vi "BCU参数读取-Auto.vi"(8 "CAN端口":u16(ring), 9 "设备索引号":u16(ring), 10 "CAN卡类型":u32(ring)=21, 11 "Myindex":dbl=1.0) -> (3 "成功":bool)   [LabVIEW 2013] (continued)
                          n1972 = global write "EV05全局变量1.vi" "流控帧 2"(FALSE ("流控帧 2")) -> ()
                          n1973 = global write "EV05全局变量1.vi" "输出数组"(i32[] []) -> ()
                          n1974 = local write "控制1"(FALSE ("控制1")) -> ()
                          n1975 = local write "消除"(FALSE ("消除")) -> ()
                        }
                      }
                    }
                    frame True {
                      # "写参数判定"
                      n1976 = And(x="控制1", y=w3317) -> (x .and. y?=w3314:bool)
                      n1977 = case shown="真" w3314 {
                        tunnel: w3316 -> [_ w3324]
                        tunnel: w3315 -> [_ w3321]
                        frame False {
                        }
                        frame True {
                          n1978 = call <vilib>:"Unset Busy.vi"() -> ()  [unwired: 2 in, 10 out]
                          n1979 = case shown="\"主板\", 默认" w3321 {
                            tunnel: [w3325 w3326] -> w3323
                            frame "主板", Default {
                              n1980 = local read "主板选项"() -> (w3325:string)
                            }
                            frame "从板" {
                              n1981 = local read "从板选项"() -> (w3326:string)
                            }
                          }
                          n1982 = control-ref of="结果"() -> (w3322:refnum<vi>)
                          n1983 = call "输入数据判定.vi"("主从选择"=w3321, "主板选项"=w3323, "进度引用"=w3322, "错误代码"=w3324) -> ()  [unwired: 3 in, 5 out]
                          n1984 = global write "EV05全局变量1.vi" "流控帧 2"(FALSE ("流控帧 2")) -> ()
                          n1985 = local write "控制1"(FALSE ("控制1")) -> ()
                          n1986 = local write "消除"(FALSE ("消除")) -> ()
                        }
                      }
                      n1987 = global write "EV05全局变量1.vi" "输出数组"(i32[] []) -> ()
                    }
                  }
                }
                frame "版本读取" {
                  n1988 = local read "命令序号"() -> (w3327:u8)
                  n1989 = local read "从板板号"() -> (w3330:u8)
                  n1990 = local read "控制1"() -> (w3331:bool)
                  n1991 = call "多帧接收机制(EV05).vi"("can卡类型"=w3338, "设备索引号"=w3337, "CAN端口"=w3336, "VCI_Receive"=w3335, "命令"=w3334, "板号"=w3330, "命令序号"=w3327) -> ("错误信号"=w3328:bool, "输出数组"=w3339:u8[], "读错误代码"=w3329:u8[], "结束信号"=w3333:bool)  [unwired: 3 in, 6 out]
                  n1992 = And(x=w3331, y=w3333) -> (x .and. y?=w3332:bool)
                  n1993 = case shown="真" w3332 {
                    tunnel: w3339 -> [_ w3347]
                    tunnel: w3327 -> [_ w3346]
                    tunnel: w3334 -> [_ w3345]
                    tunnel: w3329 -> [_ w3341]
                    tunnel: w3328 -> [_ w3340]
                    frame False {
                    }
                    frame True {
                      n1994 = case shown="假" w3340 {
                        tunnel: w3347 -> [w3351 _]
                        tunnel: w3346 -> [w3350 _]
                        tunnel: w3345 -> [w3349 _]
                        tunnel: w3341 -> [w3348 w3575]
                        frame False {
                          n1995 = case shown="89" w3349 {
                            tunnel: w3350 -> [_ w3354]
                            tunnel: w3351 -> [_ w3353]
                            tunnel: w3348 -> [_ _]
                            frame 0, Default {
                            }
                            frame 137 {
                              n1996 = case shown="1" w3354 {
                                tunnel: w3353 -> [_ w3382 w3426 w3446 w3573]
                                frame 0, Default {
                                }
                                frame 1 {
                                w3364 = "." ("字符串")
                                n1997 = Array Subset(array=w3382, index=0 ("索引"), length=14 ("长度")) -> (w3395:u8[])
                                n1998 = Index Array(array=w3382, index=14 ("索引")) -> (element=w3385:u8)
                                n1999 = Index Array(array=w3382, index #1=15 ("索引"), index #2=16 ("索引")) -> (element #1=w3391:u8, element #2=w3392:u8)
                                n2000 = Index Array(array=w3382, index #1=17 ("索引"), index #2=18 ("索引")) -> (element #1=w3386:u8, element #2=w3387:u8)
                                n2001 = call "数组去零.vi"("输入"=w3395) -> ("输出"=w3370:dbl[])
                                n2002 = Join Numbers(hi=w3386, lo=w3387) -> ((hi.lo)=w3383:u16)
                                n2003 = Join Numbers(hi=w3391, lo=w3392) -> ((hi.lo)=w3384:u16)
                                n2004 = Number To Decimal String(number=w3385) -> (decimal integer string=w3377:string)  [unwired: 1 out]
                                n2005 = Byte Array To String(unsigned byte array=w3370) -> (string=w3369:string)
                                n2006 = Number To Decimal String(number=w3383) -> (decimal integer string=w3365:string)  [unwired: 1 out]
                                n2007 = Number To Decimal String(number=w3384) -> (decimal integer string=w3376:string)  [unwired: 1 out]
                                n2008 = Array Subset(array=w3382, index=21 ("索引"), length=7 ("长度")) -> (w3379:u8[])
                                n2009 = Concatenate Strings("V" ("字符串"), w3377, w3364, w3376, w3364, w3365) -> (w3374:string)
                                n2010 = call "数组去零.vi"("输入"=w3379) -> ("输出"=w3362:dbl[])
                                n2011 = Byte Array To String(unsigned byte array=w3362) -> (string=w3360:string)
                                n2012 = call <vilib>:"Space Constant.vi"() -> ("String"=w3361:string)
                                n2013 = Equal?(x=w3360, y=w3361) -> (x = y?=w3366:bool)
                                n2014 = Concatenate Strings("-" ("字符串"), w3360) -> (w3367:string)
                                n2015 = Select(t=w3361, s=w3366, f=w3367) -> (s? t:f=w3363:string)
                                n2016 = Concatenate Strings(w3369, "-" ("字符串"), w3374, w3363) -> (w3356:string)
                                n2017 = local read "项目软件版本"() -> (w3358:string[])
                                n2018 = local read "从板板号"() -> (w3355:u8)
                                n2019 = local write "项目软件版本号"(w3356) -> ()
                                n2020 = Replace Array Subset(array=w3358, new element=w3356, index=w3355) -> (w3357:string[])
                                n2021 = control-ref of="结果"() -> (w3373:refnum<vi>)
                                n2022 = local write "项目软件版本"(w3357) -> ()
                                n2023 = Build Array("项目软件版本     读取完成" ("读取结果")) -> (w3371:string[])
                                n2024 = call "表格编辑(版本读取).vi"("新元素/子数组"=w3371, "活动单元格:单元格背景色"=u32 6618880, "MCListbox引用句柄"=w3373) -> ()  [unwired: 9 out]
                                }
                                frame 2 {
                                w3409 = ""
                                w3406 = "." ("字符串")
                                n2025 = Array Subset(array=w3426, index=0 ("索引"), length=14 ("长度")) -> (w3414:u8[])
                                n2026 = Index Array(array=w3426, index=14 ("索引")) -> (element=w3429:u8)
                                n2027 = Index Array(array=w3426, index #1=15 ("索引"), index #2=16 ("索引")) -> (element #1=w3435:u8, element #2=w3436:u8)
                                n2028 = Index Array(array=w3426, index #1=17 ("索引"), index #2=18 ("索引")) -> (element #1=w3430:u8, element #2=w3431:u8)
                                n2029 = Join Numbers(hi=w3430, lo=w3431) -> ((hi.lo)=w3427:u16)
                                n2030 = Join Numbers(hi=w3435, lo=w3436) -> ((hi.lo)=w3428:u16)
                                n2031 = Number To Decimal String(number=w3427) -> (decimal integer string=w3407:string)  [unwired: 1 out]
                                n2032 = call "数组去零.vi"("输入"=w3414) -> ("输出"=w3413:dbl[])
                                n2033 = Number To Decimal String(number=w3429) -> (decimal integer string=w3421:string)  [unwired: 1 out]
                                n2034 = Number To Decimal String(number=w3428) -> (decimal integer string=w3420:string)  [unwired: 1 out]
                                n2035 = Array Subset(array=w3426, index=21 ("索引"), length=7 ("长度")) -> (w3423:u8[])
                                n2036 = Byte Array To String(unsigned byte array=w3413) -> (string=w3408:string)
                                n2037 = call "数组去零.vi"("输入"=w3423) -> ("输出"=w3405:dbl[])
                                n2038 = Concatenate Strings("V" ("字符串"), w3421, w3406, w3420, w3406, w3407) -> (w3418:string)
                                n2039 = Byte Array To String(unsigned byte array=w3405) -> (string=w3403:string)
                                n2040 = Equal?(x=w3409, y=w3403) -> (x = y?=w3410:bool)
                                n2041 = Concatenate Strings("-" ("字符串"), w3403) -> (w3411:string)
                                n2042 = Select(t=w3409, s=w3410, f=w3411) -> (s? t:f=w3404:string)
                                n2043 = Concatenate Strings(w3408, "-" ("字符串"), w3418, w3404) -> (w3399:string)
                                n2044 = local read "平台软件版本"() -> (w3401:string[])
                                n2045 = local read "从板板号"() -> (w3398:u8)
                                n2046 = local write "平台软件版本号"(w3399) -> ()
                                n2047 = Replace Array Subset(array=w3401, new element=w3399, index=w3398) -> (w3400:string[])
                                n2048 = control-ref of="结果"() -> (w3416:refnum<vi>)
                                n2049 = local write "平台软件版本"(w3400) -> ()
                                n2050 = Build Array("平台软件版本     读取完成" ("读取结果")) -> (w3415:string[])
                                n2051 = call "表格编辑(版本读取).vi"("新元素/子数组"=w3415, "活动单元格:单元格背景色"=u32 6618880, "MCListbox引用句柄"=w3416) -> ()  [unwired: 1 in, 8 out]
                                }
                                frame 3 {
                                n2052 = Index Array(array=w3446, index #1=0 ("索引"), index #2=1 ("索引")) -> (element #1=w3442:u8, element #2=w3443:u8)
                                n2053 = Join Numbers(hi=w3442, lo=w3443) -> ((hi.lo)=w3441:u16)
                                n2054 = case shown="99, 默认" w3441 {
                                tunnel: w3446 -> [w3449 _ w3483]
                                tunnel: w3441 -> [_ _ w3461]
                                frame 0 {
                                n2055 = Index Array(array=w3449, index #1=2 ("索引"), index #2=3 ("索引")) -> (element #1=w3453:u8, element #2=w3452:u8)
                                n2056 = Join Numbers(hi=w3453, lo=w3452) -> ((hi.lo)=w3448:u16)
                                n2057 = for {
                                N: w3448 -> [_]
                                tunnel: w3449 -> [w3458]
                                tunnel: [w3454] -> w3447 mode=indexing
                                i -> [w3457]
                                n2058 = Add(x=w3457, y=4) -> (x+y=w3455:i32)
                                n2059 = Index Array(array=w3458, index=w3455) -> (element=w3454:u8)
                                }
                                "MODEL号" <- w3447
                                }
                                frame 99, Default {
                                }
                                frame 1..40 {
                                w3466 = ""
                                w3487 = "." ("字符串")
                                n2060 = Array Subset(array=w3483, index=2 ("索引"), length=14 ("长度")) -> (w3472:u8[])
                                n2061 = Index Array(array=w3483, index=16 ("索引")) -> (element=w3495:u8)
                                n2062 = Index Array(array=w3483, index #1=17 ("索引"), index #2=18 ("索引")) -> (element #1=w3501:u8, element #2=w3502:u8)
                                n2063 = Index Array(array=w3483, index #1=19 ("索引"), index #2=20 ("索引")) -> (element #1=w3496:u8, element #2=w3497:u8)
                                n2064 = Join Numbers(hi=w3496, lo=w3497) -> ((hi.lo)=w3493:u16)
                                n2065 = Join Numbers(hi=w3501, lo=w3502) -> ((hi.lo)=w3494:u16)
                                n2066 = Number To Decimal String(number=w3461) -> (decimal integer string=w3481:string)  [unwired: 1 out]
                                n2067 = Number To Decimal String(number=w3495) -> (decimal integer string=w3489:string)  [unwired: 1 out]
                                n2068 = call "数组去零.vi"("输入"=w3472) -> ("输出"=w3471:dbl[])
                                n2069 = Number To Decimal String(number=w3494) -> (decimal integer string=w3488:string)  [unwired: 1 out]
                                n2070 = Number To Decimal String(number=w3493) -> (decimal integer string=w3486:string)  [unwired: 1 out]
                                n2071 = Byte Array To String(unsigned byte array=w3471) -> (string=w3473:string)
                                n2072 = Concatenate Strings("第" ("读取结果"), w3481, "模块" ("字符串"), "     读取完成" ("读取结果")) -> (w3474:string)
                                n2073 = Concatenate Strings("V" ("字符串"), w3489, w3487, w3488, w3487, w3486) -> (w3484:string)
                                n2074 = control-ref of="结果"() -> (w3477:refnum<vi>)
                                n2075 = Array Subset(array=w3483, index=23 ("索引"), length=7 ("长度")) -> (w3470:u8[])
                                n2076 = call "数组去零.vi"("输入"=w3470) -> ("输出"=w3465:dbl[])
                                n2077 = Byte Array To String(unsigned byte array=w3465) -> (string=w3462:string)
                                n2078 = Build Array(w3474) -> (w3476:string[])
                                n2079 = control-ref of="模块软件版本 2"() -> (w3478:refnum<vi>)
                                n2080 = local read "模块软件版本"() -> (w3479:T1)
                                n2081 = Equal?(x=w3466, y=w3462) -> (x = y?=w3467:bool)
                                n2082 = call "表格编辑(版本读取).vi"("新元素/子数组"=w3476, "活动单元格:单元格背景色"=u32 6618880, "MCListbox引用句柄"=w3477) -> ()  [unwired: 1 in, 8 out]
                                n2083 = Concatenate Strings("-" ("字符串"), w3462) -> (w3468:string)
                                n2084 = Select(t=w3466, s=w3467, f=w3468) -> (s? t:f=w3464:string)
                                n2085 = Concatenate Strings(w3473, "-" ("字符串"), w3484, w3464) -> (w3463:string)
                                n2086 = case shown="30" w3461 {
                                tunnel: [_ "VERSIONM" "BCUMCAL" "BMUMCAL" "BMURMCAL" "BCUCMCAL" "BCUDMCAL" "SCH" "BSW" "CDD" "DATALAYER" "DATAANALYSIS" "SOC" "SOH" "SOF" "INTRES" "INTCAN" "CARCAN" "CHGCANL" "THM" "CHGM" "HVM" "LVM" "BALM" "SAFEM" "RUNMODEM" "RELAY" "DO" "GBCHGDET" "SUPPLYPOWGDET" "SUMVDET" "CURDET" "TEMPERDET" "CELLVDET" "ISODET" "AI" "DI" "SYSCONF" "ECUCONF"] -> w3460
                                frame 0, Default {
                                }
                                frame 1 {
                                }
                                frame 2 {
                                }
                                frame 3 {
                                }
                                frame 4 {
                                }
                                frame 5 {
                                }
                                frame 6 {
                                }
                                frame 7 {
                                }
                                frame 8 {
                                }
                                frame 9 {
                                }
                                frame 10 {
                                }
                                frame 11 {
                                }
                                frame 12 {
                                }
                                frame 13 {
                                }
                                frame 14 {
                                }
                                frame 15 {
                                }
                                frame 16 {
                                }
                                frame 17 {
                                }
                                frame 18 {
                                }
                                frame 19 {
                                }
                                frame 20 {
                                }
                                frame 21 {
                                }
                                frame 22 {
                                }
                                frame 23 {
                                }
                                frame 24 {
                                }
                                frame 25 {
                                }
                                frame 26 {
                                }
                                frame 27 {
                                }
                                frame 28 {
                                }
                                frame 29 {
                                }
                                frame 30 {
                                }
                                frame 31 {
                                }
                                frame 32 {
                                }
                                frame 33 {
                                }
                                frame 34 {
                                }
                                frame 35 {
                                }
                                frame 36 {
                                }
                                frame 37 {
                                }
                                frame 38 {
                                }
                                }
                                n2087 = case shown="\"全部读取\"" w3479 {
                                tunnel: w3463 -> [w3546 w3554]
                                tunnel: w3461 -> [w3550 w3559]
                                tunnel: w3478 -> [w3552 w3560]
                                tunnel: w3460 -> [w3551 w3558]
                                frame "全部读取" {
                                n2088 = Number To Decimal String(number=w3550) -> (decimal integer string=w3549:string)  [unwired: 1 out]
                                n2089 = Concatenate Strings(w3549, "-" ("元素"), w3551) -> (w3547:string)
                                n2090 = Build Array(w3547, w3546) -> (w3545:string[])
                                n2091 = call "表格编辑(模块版本).vi"("新元素/子数组"=w3545, "MCListbox引用句柄"=w3552) -> ()  [unwired: 1 in, 9 out]
                                }
                                frame "BCUMCAL", Default {
                                n2092 = Number To Decimal String(number=w3559) -> (decimal integer string=w3557:string)  [unwired: 1 out]
                                n2093 = Concatenate Strings(w3557, "-" ("元素"), w3558) -> (w3555:string)
                                n2094 = Build Array(w3555, w3554) -> (w3553:string[])
                                n2095 = call "表格编辑(模块版本).vi"("新元素/子数组"=w3553, "MCListbox引用句柄"=w3560) -> ()  [unwired: 1 in, 9 out]
                                }
                                }
                                }
                                }
                                }
                                frame 4 {
                                n2096 = Array Subset(array=w3573, length=12 ("长度")) -> (w3571:u8[])  [unwired: 1 in]
                                n2097 = Byte Array To String(unsigned byte array=w3571) -> (string=w3570:string)
                                n2098 = call <vilib>:"Trim Whitespace.vi"("string"=w3570) -> ("trimmed string"=w3562:string)  [unwired: 1 in]
                                n2099 = local read "从板板号"() -> (w3561:u8)
                                n2100 = local write "硬件版本号"(w3562) -> ()
                                n2101 = local read "硬件版本"() -> (w3563:string[])
                                n2102 = Replace Array Subset(array=w3563, new element=w3562, index=w3561) -> (w3564:string[])
                                n2103 = local write "硬件版本"(w3564) -> ()
                                n2104 = global write "EV05全局变量1.vi" "写入超时"(TRUE ("写入超时")) -> ()
                                n2105 = control-ref of="结果"() -> (w3568:refnum<vi>)
                                n2106 = Build Array("硬件版本     读取完成" ("读取结果")) -> (w3567:string[])
                                n2107 = call "表格编辑(版本读取).vi"("新元素/子数组"=w3567, "活动单元格:单元格背景色"=u32 6618880, "MCListbox引用句柄"=w3568) -> ()  [unwired: 9 out]
                                }
                              }
                              n2108 = global write "EV05全局变量1.vi" "写入超时"(TRUE ("写入超时")) -> ()
                            }
                          }
                        }
                        frame True {
                          n2109 = Index Array(array=w3575, index #1=0 ("索引"), index #2=1 ("索引")) -> (element #1=w3580:u8, element #2=w3581:u8)
                          n2110 = Join Numbers(hi=w3580, lo=w3581) -> ((hi.lo)=w3579:u16)
                          n2111 = Number To Hexadecimal String(2:w3579) -> (0:w3578:string)  [unwired: 1 out]
                          n2112 = control-ref of="结果"() -> (w3577:refnum<vi>)
                          n2113 = Concatenate Strings("0x" ("字符串"), w3578) -> (w3585:string)
                          n2114 = Build Array(w3585) -> (w3576:string[])
                          n2115 = call "表格编辑(版本读取).vi"("新元素/子数组"=w3576, "活动单元格:单元格背景色"=u32 16740749, "MCListbox引用句柄"=w3577) -> ()  [unwired: 9 out]
                        }
                      }
                      n2116 = global write "EV05全局变量1.vi" "流控帧 2"(FALSE ("流控帧 2")) -> ()
                      n2117 = local write "控制1"(FALSE ("控制1")) -> ()
                      n2118 = local write "消除"(FALSE ("消除")) -> ()
                      n2119 = call <vilib>:"Unset Busy.vi"() -> ()  [unwired: 2 in, 10 out]
                    }
                  }
                }
                frame "其它诊断" {
                  n2120 = local read "命令序号"() -> (w3587:u8)
                  n2121 = call "多帧接收机制(EV05).vi"("can卡类型"=w3594, "设备索引号"=w3593, "CAN端口"=w3592, "VCI_Receive"=w3591, "命令"=w3589, "板号"=w3590, "命令序号"=w3587) -> ("错误代码"=w3596:i32, "输出数组"=w3588:u8[], "读错误代码"=w3586:u8[], "结束信号"=w3595:bool)  [unwired: 3 in, 6 out]
                  n2122 = case shown="真" w3595 {
                    tunnel: w3597 -> [_ w3598]
                    tunnel: w3596 -> [_ _]
                    tunnel: w3588 -> [_ w3599]
                    tunnel: w3587 -> [_ w3602]
                    tunnel: w3586 -> [_ w3600]
                    frame False {
                    }
                    frame True {
                      n2123 = Insert Into Array(array=w3600, new element=w3599) -> (w3601:u8[])  [unwired: 1 in]
                      n2124 = case shown="1" w3602 {
                        tunnel: w3601 -> [_ w3611 w3697]
                        tunnel: w3598 -> [_ _ w3692]
                        frame 0, Default {
                        }
                        frame 1 {
                          n2125 = Index Array(array=w3611) -> (element #1=w3610:u8, element #2=w3609:u8, element #3=w3608:u8)  [unwired: 3 in]
                          n2126 = Join Numbers(hi=w3609, lo=w3608) -> ((hi.lo)=w3607:u16)
                          n2127 = case shown="4" w3610 {
                            tunnel: w3611 -> [_ _ _ _ _ _ _ _ _ _]
                            tunnel: w3607 -> [_ w3614 w3622 w3632 w3642 w3652 w3662 w3672 w3682 _]
                            frame 0, Default {
                              n2128 = local write "继电器超时处理"(FALSE ("继电器超时处理")) -> ()
                            }
                            frame 1 {
                              n2129 = Equal To 0?(x=w3614) -> (x = 0?=w3613:bool)
                              n2130 = local write "正级继电器 12"(w3613) -> ()
                              n2131 = case shown="假" w3613 {
                                tunnel: w3614 -> [w3617 _]
                                frame False {
                                n2132 = local read "正级继电器"() -> (w3619:bool)
                                n2133 = Number To Hexadecimal String(2:w3617) -> (0:w3616:string)  [unwired: 1 out]
                                n2134 = local write "继电器超时处理"(TRUE ("继电器超时处理")) -> ()
                                n2135 = Not(x=w3619) -> (.not. x?=w3618:bool)
                                n2136 = Concatenate Strings("继电器操作失败,0x" ("消息"), w3616) -> ()  [unwired: 1 out]
                                n2137 = local write "正级继电器"(w3618) -> ()
                                }
                                frame True {
                                (unwired) "继电器操作成功!\n继电器操作成功!\n继电器操作成功!"
                                }
                              }
                            }
                            frame 2 {
                              n2138 = Equal To 0?(x=w3622) -> (x = 0?=w3621:bool)
                              n2139 = case shown="假" w3621 {
                                tunnel: w3622 -> [w3628 _]
                                tunnel: [w3626 "继电器操作成功!\n继电器操作成功!\n继电器操作成功!"] -> _
                                frame False {
                                n2140 = local read "负级继电器"() -> (w3624:bool)
                                n2141 = Number To Hexadecimal String(2:w3628) -> (0:w3627:string)  [unwired: 1 out]
                                n2142 = local write "继电器超时处理"(TRUE ("继电器超时处理")) -> ()
                                n2143 = Not(x=w3624) -> (.not. x?=w3625:bool)
                                n2144 = Concatenate Strings("继电器操作失败,0x" ("消息"), w3627) -> (w3626:string)
                                n2145 = local write "负级继电器"(w3625) -> ()
                                }
                                frame True {
                                }
                              }
                              n2146 = local write "正级继电器 2"(w3621) -> ()
                            }
                            frame 3 {
                              n2147 = Equal To 0?(x=w3632) -> (x = 0?=w3631:bool)
                              n2148 = case shown="假" w3631 {
                                tunnel: w3632 -> [w3638 _]
                                tunnel: [w3636 "继电器操作成功!\n继电器操作成功!\n继电器操作成功!"] -> _
                                frame False {
                                n2149 = local read "预充电继电器"() -> (w3634:bool)
                                n2150 = Number To Hexadecimal String(2:w3638) -> (0:w3637:string)  [unwired: 1 out]
                                n2151 = local write "继电器超时处理"(TRUE ("继电器超时处理")) -> ()
                                n2152 = Not(x=w3634) -> (.not. x?=w3635:bool)
                                n2153 = Concatenate Strings("继电器操作失败,0x" ("消息"), w3637) -> (w3636:string)
                                n2154 = local write "预充电继电器"(w3635) -> ()
                                }
                                frame True {
                                }
                              }
                              n2155 = local write "正级继电器 3"(w3631) -> ()
                            }
                            frame 4 {
                              n2156 = Equal To 0?(x=w3642) -> (x = 0?=w3641:bool)
                              n2157 = case shown="假" w3641 {
                                tunnel: w3642 -> [w3648 _]
                                tunnel: [w3646 "继电器操作成功!\n继电器操作成功!\n继电器操作成功!"] -> _
                                frame False {
                                n2158 = local read "加热继电器"() -> (w3645:bool)
                                n2159 = Number To Hexadecimal String(2:w3648) -> (0:w3647:string)  [unwired: 1 out]
                                n2160 = local write "继电器超时处理"(TRUE ("继电器超时处理")) -> ()
                                n2161 = Not(x=w3645) -> (.not. x?=w3644:bool)
                                n2162 = Concatenate Strings("继电器操作失败,0x" ("消息"), w3647) -> (w3646:string)
                                n2163 = local write "加热继电器"(w3644) -> ()
                                }
                                frame True {
                                }
                              }
                              n2164 = local write "正级继电器 5"(w3641) -> ()
                            }
                            frame 5 {
                              n2165 = Equal To 0?(x=w3652) -> (x = 0?=w3651:bool)
                              n2166 = case shown="假" w3651 {
                                tunnel: w3652 -> [w3658 _]
                                tunnel: [w3656 "继电器操作成功!\n继电器操作成功!\n继电器操作成功!"] -> _
                                frame False {
                                n2167 = local read "充电继电器"() -> (w3654:bool)
                                n2168 = Number To Hexadecimal String(2:w3658) -> (0:w3657:string)  [unwired: 1 out]
                                n2169 = local write "继电器超时处理"(TRUE ("继电器超时处理")) -> ()
                                n2170 = Not(x=w3654) -> (.not. x?=w3655:bool)
                                n2171 = Concatenate Strings("继电器操作失败,0x" ("消息"), w3657) -> (w3656:string)
                                n2172 = local write "充电继电器"(w3655) -> ()
                                }
                                frame True {
                                }
                              }
                              n2173 = local write "正级继电器 4"(w3651) -> ()
                            }
                            frame 6 {
                              n2174 = Equal To 0?(x=w3662) -> (x = 0?=w3661:bool)
                              n2175 = local write "正级继电器 6"(w3661) -> ()
                              n2176 = case shown="假" w3661 {
                                tunnel: w3662 -> [w3668 _]
                                tunnel: [w3666 "继电器操作成功!\n继电器操作成功!\n继电器操作成功!"] -> _
                                frame False {
                                n2177 = local read "风机继电器"() -> (w3664:bool)
                                n2178 = Number To Hexadecimal String(2:w3668) -> (0:w3667:string)  [unwired: 1 out]
                                n2179 = local write "继电器超时处理"(TRUE ("继电器超时处理")) -> ()
                                n2180 = Not(x=w3664) -> (.not. x?=w3665:bool)
                                n2181 = Concatenate Strings("继电器操作失败,0x" ("消息"), w3667) -> (w3666:string)
                                n2182 = local write "风机继电器"(w3665) -> ()
                                }
                                frame True {
                                }
                              }
                            }
                            frame 7 {
                              n2183 = Equal To 0?(x=w3672) -> (x = 0?=w3671:bool)
                              n2184 = case shown="假" w3671 {
                                tunnel: w3672 -> [w3677 _]
                                tunnel: [w3675 "继电器操作成功!\n继电器操作成功!\n继电器操作成功!"] -> _
                                frame False {
                                n2185 = local read "加热继电器(从)"() -> (w3673:bool)
                                n2186 = Number To Hexadecimal String(2:w3677) -> (0:w3676:string)  [unwired: 1 out]
                                n2187 = Not(x=w3673) -> (.not. x?=w3674:bool)
                                n2188 = Concatenate Strings("继电器操作失败,0x" ("消息"), w3676) -> (w3675:string)
                                n2189 = local write "加热继电器(从)"(w3674) -> ()
                                }
                                frame True {
                                n2190 = local write "继电器超时处理"(TRUE ("继电器超时处理")) -> ()
                                }
                              }
                              n2191 = local write "正级继电器 7"(w3671) -> ()
                            }
                            frame 8 {
                              n2192 = Equal To 0?(x=w3682) -> (x = 0?=w3681:bool)
                              n2193 = case shown="假" w3681 {
                                tunnel: w3682 -> [w3687 _]
                                tunnel: [w3685 "继电器操作成功!\n继电器操作成功!\n继电器操作成功!"] -> _
                                frame False {
                                n2194 = local read "风机继电器(从)"() -> (w3683:bool)
                                n2195 = Number To Hexadecimal String(2:w3687) -> (0:w3686:string)  [unwired: 1 out]
                                n2196 = Not(x=w3683) -> (.not. x?=w3684:bool)
                                n2197 = Concatenate Strings("继电器操作失败,0x" ("消息"), w3686) -> (w3685:string)
                                n2198 = local write "风机继电器(从)"(w3684) -> ()
                                }
                                frame True {
                                n2199 = local write "继电器超时处理"(TRUE ("继电器超时处理")) -> ()
                                }
                              }
                              n2200 = local write "正级继电器 8"(w3681) -> ()
                            }
                            frame 85, 170 {
                              n2201 = local write "继电器超时处理"(TRUE ("继电器超时处理")) -> ()
                            }
                          }
                        }
                        frame 2 {
                          n2202 = Index Array(array=w3697) -> (element #1=w3696:u8, element #2=w3695:u8, element #3=w3694:u8)  [unwired: 3 in]
                          n2203 = Join Numbers(hi=w3695, lo=w3694) -> ((hi.lo)=w3693:u16)
                          n2204 = case shown="2" w3696 {
                            tunnel: w3697 -> [_ _ _]
                            tunnel: w3693 -> [_ w3701 w3715]
                            tunnel: w3692 -> [_ w3700 _]
                            frame 0, Default {
                              n2205 = local write "继电器超时处理"(FALSE ("继电器超时处理")) -> ()
                            }
                            frame 1 {
                              n2206 = Equal To 0?(x=w3701) -> (x = 0?=w3699:bool)
                              n2207 = case shown="假" w3699 {
                                tunnel: w3701 -> [w3707 _]
                                tunnel: [w3705 "DO控制操作成功!\nDO控制操作成功!\nDO控制操作成功!"] -> _
                                tunnel: w3700 -> [w3704 _]
                                frame False {
                                n2208 = case shown="\"主板\", 默认" w3704 {
                                frame "主板", Default {
                                n2209 = local read "DO1"() -> (w3710:bool)
                                n2210 = Not(x=w3710) -> (.not. x?=w3709:bool)
                                n2211 = local write "DO1"(w3709) -> ()
                                }
                                frame "从板" {
                                n2212 = local read "DO1 2"() -> (w3712:bool)
                                n2213 = Not(x=w3712) -> (.not. x?=w3711:bool)
                                n2214 = local write "DO1 2"(w3711) -> ()
                                }
                                }
                                n2215 = Number To Hexadecimal String(2:w3707) -> (0:w3706:string)  [unwired: 1 out]
                                n2216 = Concatenate Strings("DO控制操作失败,0x" ("消息"), w3706) -> (w3705:string)
                                }
                                frame True {
                                }
                              }
                              n2217 = case shown="\"从板\"" w3700 {
                                tunnel: w3699 -> [w3702 w3703]
                                frame "主板", Default {
                                n2218 = local write "正级继电器 9"(w3702) -> ()
                                }
                                frame "从板" {
                                n2219 = local write "正级继电器 11"(w3703) -> ()
                                }
                              }
                            }
                            frame 2 {
                              n2220 = Equal To 0?(x=w3715) -> (x = 0?=w3714:bool)
                              n2221 = case shown="假" w3714 {
                                tunnel: w3715 -> [w3720 _]
                                tunnel: [w3718 "DO控制操作成功!\nDO控制操作成功!\nDO控制操作成功!"] -> _
                                frame False {
                                n2222 = Number To Hexadecimal String(2:w3720) -> (0:w3719:string)  [unwired: 1 out]
                                n2223 = local read "DO2"() -> (w3717:bool)
                                n2224 = Not(x=w3717) -> (.not. x?=w3716:bool)
                                n2225 = Concatenate Strings("DO控制操作失败,0x" ("消息"), w3719) -> (w3718:string)
                                n2226 = local write "DO2"(w3716) -> ()
                                }
                                frame True {
                                }
                              }
                              n2227 = local write "正级继电器 10"(w3714) -> ()
                            }
                          }
                        }
                      }
                      n2228 = local write "消除"(FALSE ("消除")) -> ()
                      n2229 = global write "EV05全局变量1.vi" "流控帧 2"(FALSE ("流控帧 2")) -> ()
                      n2230 = local write "控制1"(FALSE ("控制1")) -> ()
                      "继电器超时处理" <- TRUE ("控制1")
                    }
                  }
                }
                frame "高压板校正" {
                  n2231 = local read "命令序号"() -> (w3727:u8)
                  n2232 = call "多帧接收机制(EV05).vi"("can卡类型"=w3734, "设备索引号"=w3733, "CAN端口"=w3732, "VCI_Receive"=w3731, "命令"=w3729, "板号"=w3730, "命令序号"=w3727) -> ("错误信号"=w3723:bool, "错误代码"=w3736:i32, "输出数组"=w3728:u8[], "读错误代码"=w3726:u8[], "结束信号"=w3735:bool)  [unwired: 3 in, 5 out]
                  n2233 = local read "控制1"() -> (w3724:bool)
                  n2234 = And(x=w3724, y=w3735) -> (x .and. y?=w3725:bool)
                  n2235 = case shown="真" w3725 {
                    tunnel: w3737 -> [_ w3741]
                    tunnel: w3736 -> [_ _]
                    tunnel: w3728 -> [_ w3739]
                    tunnel: w3727 -> [_ w3740]
                    tunnel: w3726 -> [_ w3742]
                    tunnel: w3723 -> [_ w3743]
                    frame False {
                    }
                    frame True {
                      n2236 = case shown="假" w3743 {
                        tunnel: w3742 -> [_ w3953]
                        tunnel: w3741 -> [_ _]
                        tunnel: w3740 -> [w3748 _]
                        tunnel: w3739 -> [w3747 _]
                        frame False {
                          n2237 = case shown="2" w3748 {
                            tunnel: w3747 -> [_ w3753 w3787 w3817 w3844 w3871 w3898 w3925]
                            frame 0, Default {
                            }
                            frame 1 {
                              n2238 = for {
                                N: 10 -> [_]
                                tunnel: w3753 -> [w3770]
                                shift-right: [w3757] -> w3751
                                shift-left: string[] [] -> [w3759]
                                i -> [w3756]
                                w3764 = 8 ("索引")
                                w3768 = 2 ("y")
                                n2239 = Multiply(x=w3756, y=w3768) -> (x*y=w3769:i32)
                                n2240 = Array Subset(array=w3770, index=w3769, length=w3768) -> (w3767:u8[])
                                n2241 = Index Array(array=w3767) -> (element #1=w3766:u8, element #2=w3765:u8)  [unwired: 2 in]
                                n2242 = call "二进制解析-8.6.vi"("索引"=w3764, "数值"=w3766) -> ("低位子数组"=w3763:i32[])  [unwired: 1 in, 2 out]
                                n2243 = call "二进制解析-8.6.vi"("索引"=w3764, "数值"=w3765) -> ("低位子数组"=w3762:i32[])  [unwired: 1 in, 2 out]
                                n2244 = Insert Into Array(array=w3763, new element=w3762) -> (w3761:i32[])  [unwired: 1 in]
                                n2245 = case shown="2" w3756 {
                                tunnel: [6 15 9 4 2 0 2] -> w3755
                                frame 0, Default {
                                }
                                frame 1 {
                                }
                                frame 2 {
                                }
                                frame 3..5 {
                                }
                                frame 8, 9 {
                                }
                                frame 7 {
                                }
                                frame 6 {
                                }
                                }
                                n2246 = Reverse 1D Array(array=w3761) -> (reversed array=w3760:i32[])
                                n2247 = for {
                                N: w3755 -> [_]
                                tunnel: w3760 -> [w3782] mode=indexing
                                tunnel: [w3778] -> w3758 mode=indexing
                                n2248 = Equal To 0?(x=w3782) -> (x = 0?=w3781:bool)
                                n2249 = Select(t="无", s=w3781, f="故障") -> (s? t:f=w3778:string)
                                }
                                n2250 = Insert Into Array(array=w3759, new element=w3758) -> (w3757:string[])  [unwired: 1 in]
                              }
                              n2251 = call "详细故障分解.vi"("名称"=string[] ["上电自检异常(CellV)", "通讯异常(CellV)", "不更新(CellV)", "未校准(CellV)", "保留", "采样线路断路(CellV)", "18b20上电自检异常(T) ", "18b20通讯异常(T)", "18b20传感器丢失(T)", "18b20传感器无号(T)", "18b20温度异常跳变(T)", "18b20信号线对电源短路(T)", "18b20信号线对地短路(T)", "18b20 CRC校验异常(T)", "NTC上电自检异常(T)", "NTC通讯异常(T)", "NTC传感器丢失(T)", "NTC温度异常跳变(T)", "NTC信号线断路(T)", "NTC信号线对电源短(T)", "NTC信号线对地短路(T)", "上电自检异常(Curr)", "参数异常(Curr)", "不更新(Curr)", "未校准(Curr)", "采样线断开(Curr)", "电流零漂异常(Curr)", "传感器反接(Curr)", "读取实时电流故障(Curr)", "平均电流故障(Curr)", "自检异常(iso)", "前端检测电阻损坏(iso)", "不更新(iso)", "未校准(iso)", "上电自检异常(Sumv_in)", "通讯异常(Sumv_in)", "不更新(Sumv_in)", "未校准(Sumv_in)", "上电自检异常(Sumv_out)", "通讯异常(Sumv_out)", "不更新(Sumv_out)", "未校准(Sumv_out)", "系统时钟自检异常(Clock)", "系统时钟未校准(Clock)", "充电均衡模块不能开启", "充电均衡模块不能关闭", "放电均衡模块不能开启", "放电均衡模块不能关闭"], "故障输入口"=w3751) -> ("输出数组"=w3749:string[][])  [unwired: 1 in, 2 out]
                              n2252 = local write "电池故障"(w3749) -> ()
                            }
                            frame 2 {
                              n2253 = for {
                                N: 5 -> [_]
                                tunnel: w3787 -> [w3804]
                                shift-right: [w3791] -> w3785
                                shift-left: string[] [] -> [w3793]
                                i -> [w3789]
                                w3798 = 8 ("索引")
                                w3802 = 2 ("y")
                                n2254 = Multiply(x=w3789, y=w3802) -> (x*y=w3803:i32)
                                n2255 = Array Subset(array=w3804, index=w3803, length=w3802) -> (w3801:u8[])
                                n2256 = Index Array(array=w3801) -> (element #1=w3800:u8, element #2=w3799:u8)  [unwired: 2 in]
                                n2257 = call "二进制解析-8.6.vi"("索引"=w3798, "数值"=w3800) -> ("低位子数组"=w3797:i32[])  [unwired: 1 in, 2 out]
                                n2258 = call "二进制解析-8.6.vi"("索引"=w3798, "数值"=w3799) -> ("低位子数组"=w3796:i32[])  [unwired: 1 in, 2 out]
                                n2259 = Insert Into Array(array=w3797, new element=w3796) -> (w3795:i32[])  [unwired: 1 in]
                                n2260 = case shown="2" w3789 {
                                tunnel: [4 6 5] -> w3790
                                frame 0, Default {
                                }
                                frame 2 {
                                }
                                frame 4 {
                                }
                                }
                                n2261 = Reverse 1D Array(array=w3795) -> (reversed array=w3794:i32[])
                                n2262 = for {
                                N: w3790 -> [_]
                                tunnel: w3794 -> [w3812] mode=indexing
                                tunnel: [w3808] -> w3792 mode=indexing
                                n2263 = Equal To 0?(x=w3812) -> (x = 0?=w3811:bool)
                                n2264 = Select(t="无", s=w3811, f="故障") -> (s? t:f=w3808:string)
                                }
                                n2265 = Insert Into Array(array=w3793, new element=w3792) -> (w3791:string[])  [unwired: 1 in]
                              }
                              n2266 = call "详细故障分解.vi"("名称"=string[] ["自检异常(ee_cpu)", "存储空间满(ee_cpu)", "数据写入失败(ee_cpu)", "数据读取异常(ee_cpu)", "自检异常(ee_ext)", "存储空间满(ee_ext)", "数据写入失败(ee_ext)", "数据读取异常(ee_ext)", "自检异常(flash_ext)", "故障数据存储空间满(flash_ext)", "历史数据存储空间满(flash_ext)", "数据写入失败(flash_ext)", "数据读取失败(flash_ext)", "数据校验异常(flash_ext)", "自检异常(flash_cpu)", "存储空间满(flash_cpu)", "数据写入失败(flash_cpu)", "数据读取异常(flash_cpu)", "应用程序异常(cpu)", "应用程序下载异常(cpu)", "AD模块异常(cpu)", "RAM异常(cpu)", "CPU异常下电(cpu)"], "故障输入口"=w3785) -> ("输出数组"=w3783:string[][])  [unwired: 1 in, 2 out]
                              n2267 = local write "电池故障"(w3783) -> ()
                            }
                            frame 3 {
                              n2268 = for {
                                N: 5 -> [_]
                                tunnel: w3817 -> [w3834]
                                shift-right: [w3821] -> w3815
                                shift-left: string[] [] -> [w3823]
                                i -> [w3820]
                                w3828 = 8 ("索引")
                                w3832 = 2 ("y")
                                n2269 = Multiply(x=w3820, y=w3832) -> (x*y=w3833:i32)
                                n2270 = Array Subset(array=w3834, index=w3833, length=w3832) -> (w3831:u8[])
                                n2271 = Index Array(array=w3831) -> (element #1=w3830:u8, element #2=w3829:u8)  [unwired: 2 in]
                                n2272 = call "二进制解析-8.6.vi"("索引"=w3828, "数值"=w3830) -> ("低位子数组"=w3827:i32[])  [unwired: 1 in, 2 out]
                                n2273 = call "二进制解析-8.6.vi"("索引"=w3828, "数值"=w3829) -> ("低位子数组"=w3826:i32[])  [unwired: 1 in, 2 out]
                                n2274 = Insert Into Array(array=w3827, new element=w3826) -> (w3825:i32[])  [unwired: 1 in]
                                n2275 = Reverse 1D Array(array=w3825) -> (reversed array=w3824:i32[])
                                n2276 = for {
                                N: 6 -> [_]
                                tunnel: w3824 -> [w3839] mode=indexing
                                tunnel: [w3835] -> w3822 mode=indexing
                                n2277 = Equal To 0?(x=w3839) -> (x = 0?=w3838:bool)
                                n2278 = Select(t="无", s=w3838, f="故障") -> (s? t:f=w3835:string)
                                }
                                n2279 = Insert Into Array(array=w3823, new element=w3822) -> (w3821:string[])  [unwired: 1 in]
                              }
                              n2280 = call "详细故障分解.vi"("名称"=string[] ["初始化失败(CAN4)", "发送异常(CAN4)", "接收异常(CAN4)", "总线超时(CAN4)", "BUSOFF(CAN4)", "帧格式(CAN4)", "初始化异常(CAN0)", "发送异常(CAN0)", "接收异常(CAN0)", "总线超时(CAN0)", "BUSOFF(CAN0)", "帧格式(CAN0)", "初始化异常(CAN1)", "发送异常(CAN1)", "接收异常(CAN1)", "总线超时(CAN1)", "BUSOFF(CAN1)", "帧格式(CAN1)", "初始化失败(CAN2)", "发送异常(CAN2)", "接收异常(CAN2)", "总线超时(CAN2)", "BUSOFF(CAN2)", "帧格式(CAN2)", "初始化失败(CAN3)", "发送异常(CAN3)", "接收异常(CAN3)", "总线超时(CAN3)", "BUSOFF(CAN3)", "帧格式(CAN3)"], "故障输入口"=w3815) -> ("输出数组"=w3813:string[][])  [unwired: 1 in, 2 out]
                              n2281 = local write "电池故障"(w3813) -> ()
                            }
                            frame 4 {
                              n2282 = for {
                                N: 1 -> [_]
                                tunnel: w3844 -> [w3861]
                                shift-right: [w3848] -> w3842
                                shift-left: string[] [] -> [w3850]
                                i -> [w3847]
                                w3855 = 8 ("索引")
                                w3859 = 2 ("y")
                                n2283 = Multiply(x=w3847, y=w3859) -> (x*y=w3860:i32)
                                n2284 = Array Subset(array=w3861, index=w3860, length=w3859) -> (w3858:u8[])
                                n2285 = Index Array(array=w3858) -> (element #1=w3857:u8, element #2=w3856:u8)  [unwired: 2 in]
                                n2286 = call "二进制解析-8.6.vi"("索引"=w3855, "数值"=w3857) -> ("低位子数组"=w3854:i32[])  [unwired: 1 in, 2 out]
                                n2287 = call "二进制解析-8.6.vi"("索引"=w3855, "数值"=w3856) -> ("低位子数组"=w3853:i32[])  [unwired: 1 in, 2 out]
                                n2288 = Insert Into Array(array=w3854, new element=w3853) -> (w3852:i32[])  [unwired: 1 in]
                                n2289 = Reverse 1D Array(array=w3852) -> (reversed array=w3851:i32[])
                                n2290 = for {
                                N: 4 -> [_]
                                tunnel: w3851 -> [w3866] mode=indexing
                                tunnel: [w3862] -> w3849 mode=indexing
                                n2291 = Equal To 0?(x=w3866) -> (x = 0?=w3865:bool)
                                n2292 = Select(t="无", s=w3865, f="故障") -> (s? t:f=w3862:string)
                                }
                                n2293 = Insert Into Array(array=w3850, new element=w3849) -> (w3848:string[])  [unwired: 1 in]
                              }
                              n2294 = call "详细故障分解.vi"("名称"=string[] ["通讯协议版本不一致(soft)", "系统不同步(soft)", "软件版本不一致(soft)", "同硬件平台不兼容(soft)"], "故障输入口"=w3842) -> ("输出数组"=w3840:string[][])  [unwired: 1 in, 2 out]
                              n2295 = local write "电池故障"(w3840) -> ()
                            }
                            frame 5 {
                              n2296 = for {
                                N: 2 -> [_]
                                tunnel: w3871 -> [w3888]
                                shift-right: [w3875] -> w3869
                                shift-left: string[] [] -> [w3877]
                                i -> [w3874]
                                w3882 = 8 ("索引")
                                w3886 = 2 ("y")
                                n2297 = Multiply(x=w3874, y=w3886) -> (x*y=w3887:i32)
                                n2298 = Array Subset(array=w3888, index=w3887, length=w3886) -> (w3885:u8[])
                                n2299 = Index Array(array=w3885) -> (element #1=w3884:u8, element #2=w3883:u8)  [unwired: 2 in]
                                n2300 = call "二进制解析-8.6.vi"("索引"=w3882, "数值"=w3884) -> ("低位子数组"=w3881:i32[])  [unwired: 1 in, 2 out]
                                n2301 = call "二进制解析-8.6.vi"("索引"=w3882, "数值"=w3883) -> ("低位子数组"=w3880:i32[])  [unwired: 1 in, 2 out]
                                n2302 = Insert Into Array(array=w3881, new element=w3880) -> (w3879:i32[])  [unwired: 1 in]
                                n2303 = Reverse 1D Array(array=w3879) -> (reversed array=w3878:i32[])
                                n2304 = for {
                                N: 4 -> [_]
                                tunnel: w3878 -> [w3893] mode=indexing
                                tunnel: [w3889] -> w3876 mode=indexing
                                n2305 = Equal To 0?(x=w3893) -> (x = 0?=w3892:bool)
                                n2306 = Select(t="无", s=w3892, f="故障") -> (s? t:f=w3889:string)
                                }
                                n2307 = Insert Into Array(array=w3877, new element=w3876) -> (w3875:string[])  [unwired: 1 in]
                              }
                              n2308 = call "详细故障分解.vi"("名称"=string[] ["初始化失败(RS232)", "发送异常(RS232)", "接收异常(RS232)", "总线超时(RS232)", "初始化失败(RS485)", "发送异常(RS485)", "接收异常(RS485)", "总线超时(RS485)"], "故障输入口"=w3869) -> ("输出数组"=w3867:string[][])  [unwired: 1 in, 2 out]
                              n2309 = local write "电池故障"(w3867) -> ()
                            }
                            frame 6 {
                              n2310 = for {
                                N: 2 -> [_]
                                tunnel: w3898 -> [w3915]
                                shift-right: [w3902] -> w3896
                                shift-left: string[] [] -> [w3904]
                                i -> [w3901]
                                w3909 = 8 ("索引")
                                w3913 = 2 ("y")
                                n2311 = Multiply(x=w3901, y=w3913) -> (x*y=w3914:i32)
                                n2312 = Array Subset(array=w3915, index=w3914, length=w3913) -> (w3912:u8[])
                                n2313 = Index Array(array=w3912) -> (element #1=w3911:u8, element #2=w3910:u8)  [unwired: 2 in]
                                n2314 = call "二进制解析-8.6.vi"("索引"=w3909, "数值"=w3911) -> ("低位子数组"=w3908:i32[])  [unwired: 1 in, 2 out]
                                n2315 = call "二进制解析-8.6.vi"("索引"=w3909, "数值"=w3910) -> ("低位子数组"=w3907:i32[])  [unwired: 1 in, 2 out]
                                n2316 = Insert Into Array(array=w3908, new element=w3907) -> (w3906:i32[])  [unwired: 1 in]
                                n2317 = Reverse 1D Array(array=w3906) -> (reversed array=w3905:i32[])
                                n2318 = for {
                                N: 16 -> [_]
                                tunnel: w3905 -> [w3920] mode=indexing
                                tunnel: [w3916] -> w3903 mode=indexing
                                n2319 = Equal To 0?(x=w3920) -> (x = 0?=w3919:bool)
                                n2320 = Select(t="无", s=w3919, f="故障") -> (s? t:f=w3916:string)
                                }
                                n2321 = Insert Into Array(array=w3904, new element=w3903) -> (w3902:string[])  [unwired: 1 in]
                              }
                              n2322 = call "详细故障分解.vi"("名称"=string[] ["DI1对地短", "DI1对电源短", "DI2对地短", "DI2对电源短", "DI3对地短", "DI3对电源短", "DI4对地短", "DI4对电源短", "DI5对地短", "DI5对电源短", "DI6对地短", "DI6对电源短", "DI7对地短", "DI7对电源短", "DI8对地短", "DI8对电源短", "DO1对地短", "DO1对电源短", "DO2对地短", "DO2对电源短", "DO3对地短", "DO3对电源短", "DO4对地短", "DO4对电源短", "DO5对地短", "DO5对电源短", "DO6对地短", "DO6对电源短", "DO7对地短", "DO7对电源短", "DO8对地短", "DO8对电源短"], "故障输入口"=w3896) -> ("输出数组"=w3894:string[][])  [unwired: 1 in, 2 out]
                              n2323 = local write "电池故障"(w3894) -> ()
                            }
                            frame 7 {
                              n2324 = for {
                                N: 2 -> [_]
                                tunnel: w3925 -> [w3942]
